vi "Main Flir-Ax8.vi"() -> ()   [LabVIEW 2016]
uses:
  X-Control/Run.xctl
  <vilib>/vision/Image Controls.llb/IMAQ Image.ctl
  Global Flir-Ax8.vi
  <vilib>/httpClient/LabVIEWHTTPClient.lvlib
panel:
  out "live temperature":dbl format="%#_3g"
  out "Active":bool
  in  "Tab Control":enum32{"initialize", "Thermal", "Data"}(tab)
  in  "Password :":string="admin"
  in  "User Name :":string="admin"
  in  "IP Address :":string="169.254.60.23"
  in  "File name & format :":string="Thermal.csv"
  in  "Image Folder :":path=path "C:/Users/Matanel/Desktop/Final Project/project versions/Flir-Ax8"
  in  "Run":dbl(xcontrol)
  out "Image":T1(plugin-control)
  in  "Stop":bool
  out "High Temperature":bool
  out "Temperature In Range":bool
  in  "Take image":bool
  out "Temperature":cluster{dbl, dbl, dbl, dbl, dbl}(slide)={0.0, 12.0, 13.0, 0.0, 0.0} scale=0.0..60.0 scale format="%#_3g"
  in  "Temperature Limit":dbl=60.0
  in  "Min Temperature":dbl=15.0
  in  "Max Temperature":dbl=60.0
  out "Communication":bool
  in  "Reset":bool
  in  "Table":string[][](table)
  # "Flir-Ax8 Thermal Image"
  # "11"
  # "8"
  # "1"
  # "1"
  # "3"
  # "4"
  # "3"
  # "6"
  # "1"
  # "2"
  # "1"
  # "4"
  # "Login"
  # "Initialize Data"
  # "9"
  # "10"
  # "5"
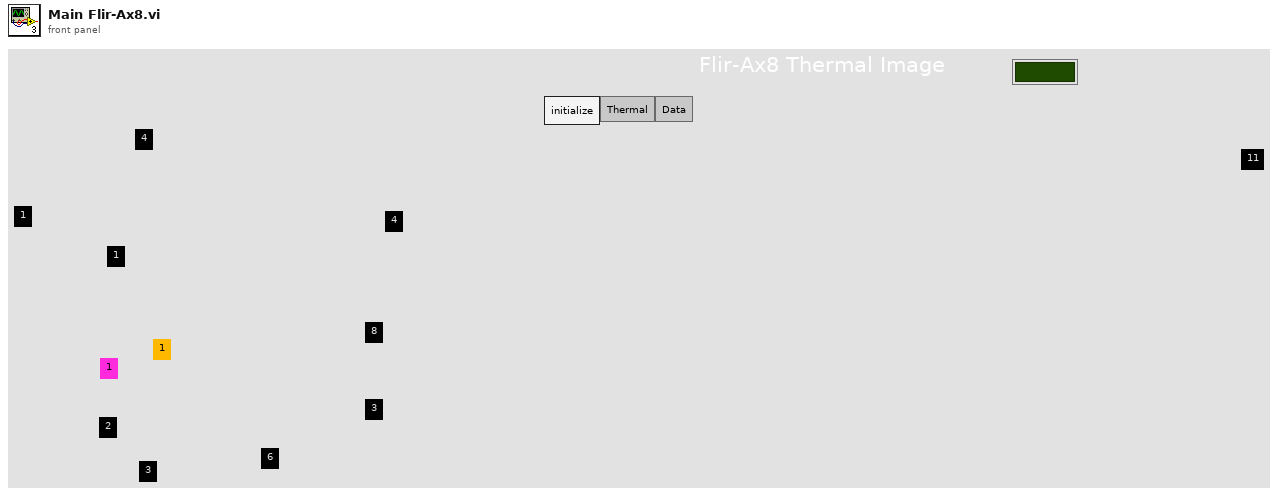
[diagram p1: front panel]
types:
  T1 = typedef "IMAQ Image.ctl" = refnum<image>
  T2 = enum8{"Enabled", "Disabled", "Disabled and Grayed Out"}
  T3 = typedef "imagedata.ctl" = cluster{"image type":i32, "image depth":i32, "image":u8[], "mask":u8[], "colors":u32[], "Rectangle":cluster{"left":i16, "top":i16, "right":i16, "bottom":i16}}
  T4 = typedef "Image Type" = u32
  T5 = typedef "LabVIEWHTTPClient.lvlib/ClientHandle.ctl" = refnum<k1>
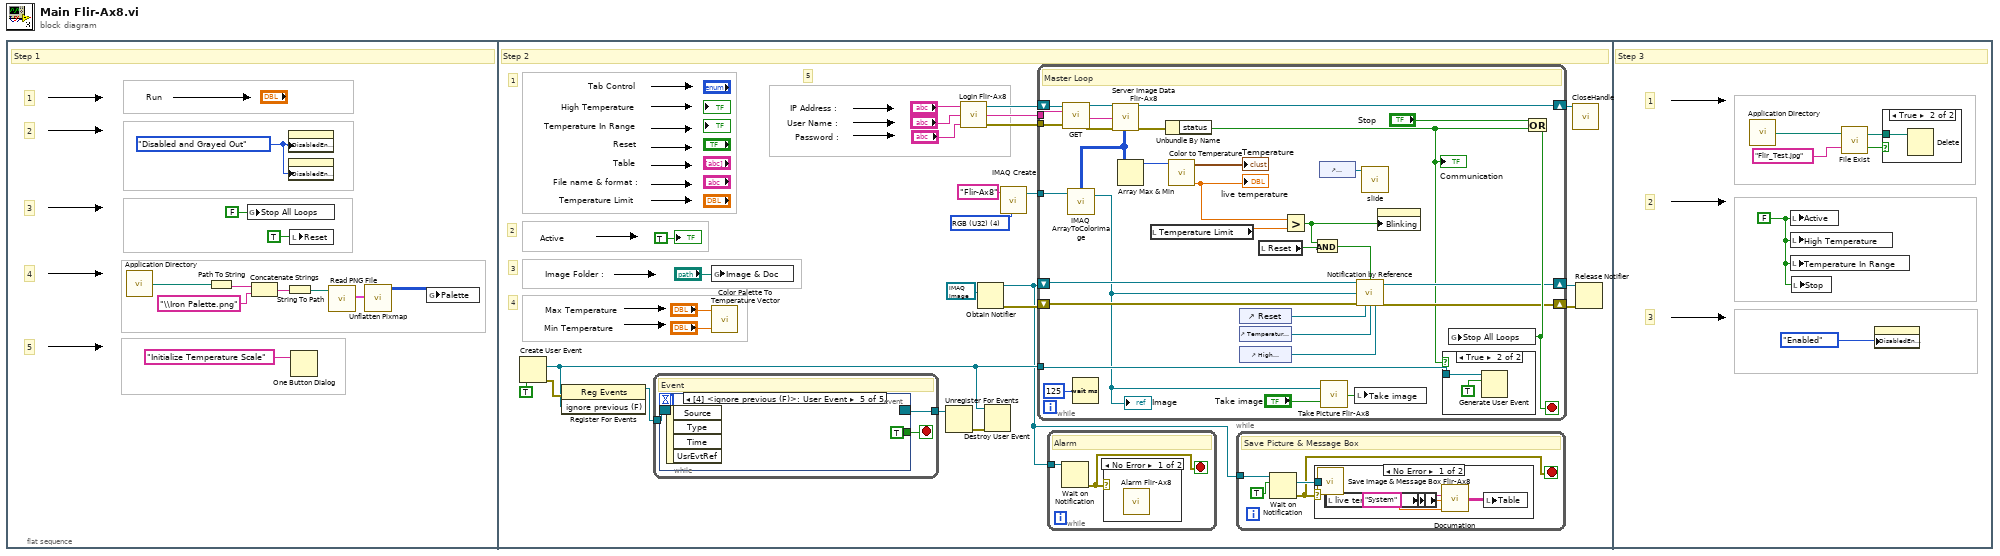
[diagram p0: block diagram]
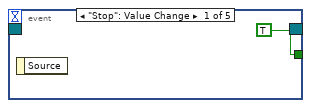
[diagram p2: hidden frame]
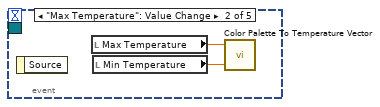
[diagram p3: hidden frame]
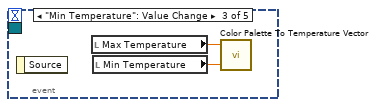
[diagram p4: hidden frame]
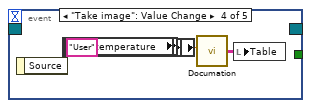
[diagram p5: hidden frame]
diagram:
  n1 = flat-sequence {
    frame #0 {
      w1 = T2."Disabled and Grayed Out" ("Disabled")
      # "5"
      # "4"
      # "3"
      # "2"
      # "1"
      # "Step 1"
      n2 = call <vilib>:"Application Directory.vi"() -> ("Application Directory"=w2:path)
      n3 = Path To String(path=w2) -> (string=w6:string)
      n4 = global write "Global Flir-Ax8.vi" "Stop All Loops"(FALSE ("Stop All Loops")) -> ()
      n5 = Concatenate Strings ("add")(w6, "\\Iron Palette.png" ("string")) -> (w5:string)
      n6 = String To Path(string=w5) -> (path=w4:path)
      n7 = property on="Run" class="Run (strict)"("DisabledEnum"=w1) -> ()  [unwired: 2 in, 2 out]
      n8 = property on="Reset" class="Bool (strict)"("DisabledEnum"=w1) -> ()  [unwired: 2 in, 2 out]
      n9 = local write "Reset"(TRUE ("Reset")) -> ()
      n10 = One Button Dialog(message="Initialize Temperature Scale") -> ()  [unwired: 1 in, 1 out]
      n11 = call <vilib>:"Read PNG File.vi"("path to PNG file"=w4) -> ("image data"=w10:T3)  [unwired: 8 in, 2 out]
      n12 = call <vilib>:"Unflatten Pixmap.vi"("image data"=w10) -> ("24-bit pixmap"=w11:u32[][])  [unwired: 4 in, 6 out]
      n13 = global write "Global Flir-Ax8.vi" "Palette"(w11) -> ()
    }
    frame #1 {
      w35 = T4 4 items=["Grayscale (U8)", "Grayscale (I16)", "Grayscale (SGL)", "Complex (CSG)", "RGB (U32)", "HSL (U32)", "RGB (U64)", "Grayscale (U16)"] ("Image Type")
      # "5"
      # "4"
      # "3"
      # "2"
      # "1"
      # "Step 2"
      n14 = Create User Event(user event datatype=TRUE ("ignore previous (F)")) -> (user event=w13:refnum<user-event>, error out=w23:errorcluster)  [unwired: 1 in]
      n15 = register-events(error in=w23, w13) -> (reference out=w21:refnum<event-registration>)  [unwired: 1 in, 1 out]
      n16 = while {
        tunnel: w21 -> [w39]
        tunnel: [w38] -> w20
        stop <- w37 stop-if-true
        # "Event"
        n17 = event shown="[4] <ignore previous (F)>: User Event" {
          selector: w39 -> [_ _ _ _ _]
          dyn-events: [_ _ _ _ _] -> w38
          timeout: _ -> [_ _ _ _ _]
          tunnel: [TRUE ("Active") _ _ _ TRUE ("Active")] -> w37
          event "Stop": Value Change {
            n18 = event-data() -> ()  [unwired: 1 in, 1 out]
          }
          event "Max Temperature": Value Change {
            n19 = event-data() -> ()  [unwired: 1 in, 1 out]
            n20 = local read "Max Temperature"() -> (w42:dbl)
            n21 = local read "Min Temperature"() -> (w41:dbl)
            n22 = call "Color Palette To Temperature Vector.vi"("Min Temperature"=w41, "Max Temperature"=w42) -> ()  [unwired: 3 in]
          }
          event "Min Temperature": Value Change {
            n23 = event-data() -> ()  [unwired: 1 in, 1 out]
            n24 = local read "Max Temperature"() -> (w44:dbl)
            n25 = local read "Min Temperature"() -> (w43:dbl)
            n26 = call "Color Palette To Temperature Vector.vi"("Min Temperature"=w43, "Max Temperature"=w44) -> ()  [unwired: 3 in]
          }
          event "Take image": Value Change {
            n27 = event-data() -> ()  [unwired: 1 in, 1 out]
            n28 = local read "Min Temperature"() -> (w49:dbl)
            n29 = local read "File name & format :"() -> (w46:string)
            n30 = local read "live temperature"() -> (w47:dbl)
            n31 = local read "Max Temperature"() -> (w50:dbl)
            n32 = call "Documation.vi"("Max Scale"=w50, "File Nm and format"=w46, "User/System"="User" ("File Nm and format"), "Temp"=w47, "Min Scale"=w49) -> ("Table"=w45:string[][])
            n33 = local write "Table"(w45) -> ()
          }
          event User Event {
            n34 = event-data() -> ()  [unwired: 1 in, 4 out]
          }
        }
      }
      n35 = global write "Global Flir-Ax8.vi" "Image & Doc"("Image Folder :") -> ()
      n36 = call "Color Palette To Temperature Vector.vi"("Min Temperature"="Min Temperature", "Max Temperature"="Max Temperature") -> ()  [unwired: 3 in]
      n37 = Unregister For Events(event registration refnum=w20) -> (error out=w19:errorcluster)  [unwired: 1 in]
      n38 = call "Login Flir-Ax8.vi"("Password"="Password :", "User Name"="User Name :", "IP"="IP Address :") -> ("Error"=w24:errorcluster, "Image Request"=w31:string, "Client Handle"=w32:T5)
      n39 = Obtain Notifier(notification data type=T1 refnum ("Image Out")) -> (notifier out=w12:refnum<notifier>, error out=w18:errorcluster)  [unwired: 2 in, 2 out]
      n40 = Destroy User Event(user event=w13, error in=w19) -> ()  [unwired: 1 out]
      n41 = call "IMAQ Create"("Image Name"="Flir-Ax8", "Image Type"=w35) -> ("New Image"=w33:T1)  [unwired: 3 in, 1 out]
      n42 = while {
        shift-right: [w81] -> w26
        shift-left: w18 -> [w79]
        shift-right: [w82] -> w27
        shift-left: w12 -> [w80]
        shift-right: [w94] -> w25
        shift-left: w32 -> [w95]
        tunnel: w33 -> [w93]
        tunnel: w31 -> [w92]
        tunnel: w24 -> [w88]
        tunnel: w13 -> [w68]
        stop <- w83 stop-if-true
        # "Master Loop"
        n43 = call <vilib>:"GET.vi"("client handle"=w95, "url"=w92, "error in (no error)"=w88) -> ("client handle out"=w94:T5, "body"=w73:string, "error out"=w72:errorcluster)  [unwired: 9 in, 1 out]
        n44 = Wait (ms)(milliseconds to wait=u32 125) -> ()  [unwired: 1 out]
        n45 = call "Server Image Data Flir-Ax8.vi"("Server Data"=w73, "Error In"=w72) -> ("Image matrix out"=w86:u32[][], "Error Out"=w87:errorcluster)  [unwired: 12 in]
        n46 = call "IMAQ ArrayToColorImage"("Image Pixels (U32)"=w86, "Image"=w93) -> ("Image Out"=w67:T1)  [unwired: 3 in, 1 out]
        "Image" <- w67
        n47 = Array Max & Min(array=w86) -> (max value=w74:u32)  [unwired: 3 out]
        n48 = local read "Temperature Limit"() -> (w85:dbl)
        n49 = Unbundle By Name(w87) -> ("status"=w65:bool)
        "Communication" <- w65
        n50 = call "Color to Temperature.vi"("Color"=w74) -> ("Temperature"=w70:dbl, "Slide"=→"Temperature":cluster{dbl, dbl, dbl, dbl, dbl})  [unwired: 7 in]
        "live temperature" <- w70
        n51 = control-ref of="Reset"() -> (w77:refnum<vi>)
        n52 = control-ref of="Temperature In Range"() -> (w76:refnum<vi>)
        n53 = control-ref of="High Temperature"() -> (w75:refnum<vi>)
        n54 = local read "Reset"() -> (w84:bool)
        n55 = Greater?(x=w70, y=w85) -> (0:w69:bool)
        n56 = And(x=w69, y=w84) -> (x .and. y?=w78:bool)
        n57 = control-ref of="Temperature"() -> (w90:refnum<vi>)
        n58 = call "Take Picture Flir-Ax8.vi"("Take Picture"="Take image", "Image"=w67) -> ("Reset Button"=w89:bool)
        n59 = local write "Take image"(w89) -> ()
        n60 = call "Notification by Reference.vi"("Notifier In"=w80, "Temperature & Reset"=w78, "Image In"=w67, "Error In"=w79, "Reset"=w77, "Temperature In Range"=w76, "High Temperature"=w75) -> ("Notifier out"=w82:refnum<notifier>, "Error out"=w81:errorcluster)  [unwired: 7 in]
        n61 = call "slide.vi"("Slide in"=w90) -> ()  [unwired: 11 in]
        n62 = property on="Temperature" class="Slide (strict)"("Blinking"=w69) -> ()  [unwired: 2 in, 2 out]
        n63 = case shown="True" w65 {
          tunnel: w68 -> [_ w97]
          frame False {
          }
          frame True {
            n64 = Generate User Event(user event=w97, event data cluster=TRUE ("ignore previous (F)")) -> ()  [unwired: 2 in, 2 out]
          }
        }
        n65 = Or(x="Stop", y=w65) -> (x .or. y?=w83:bool)
        n66 = global write "Global Flir-Ax8.vi" "Stop All Loops"(w83) -> ()
      }
      n67 = while {
        tunnel: w12 -> [w63]
        stop <- w64 stop-if-true
        # "Alarm"
        n68 = Wait on Notification(notifier=w63) -> (error out=w64:errorcluster)  [unwired: 1 in, 5 out]
        n69 = case shown="No Error" w64 {
          frame No Error {
            n70 = call "Alarm Flir-Ax8.vi"() -> ()  [unwired: 2 in]
          }
          frame Error {
          }
        }
      }
      n71 = while {
        tunnel: w12 -> [w52]
        stop <- w53 stop-if-true
        # "Save Picture & Message Box"
        n72 = Wait on Notification(notifier=w52, ignore previous (F)=TRUE) -> (notification=w55:T1, error out=w53:errorcluster)  [unwired: 1 in, 3 out]
        n73 = case shown="No Error" w53 {
          tunnel: w55 -> [w62 _]
          frame No Error {
            n74 = call "Save Image & Message Box Flir-Ax8.vi"("Image"=w62) -> ()  [unwired: 1 in]
            n75 = local read "File name & format :"() -> (w57:string)
            n76 = local read "Max Temperature"() -> (w60:dbl)
            n77 = local read "live temperature"() -> (w61:dbl)
            n78 = local read "Min Temperature"() -> (w59:dbl)
            n79 = call "Documation.vi"("Max Scale"=w60, "File Nm and format"=w57, "User/System"="System" ("File Nm and format"), "Temp"=w61, "Min Scale"=w59) -> ("Table"=w56:string[][])
            n80 = local write "Table"(w56) -> ()
          }
          frame Error {
          }
        }
      }
      n81 = call <vilib>:"CloseHandle.vi"("client handle"=w25) -> ()  [unwired: 14 in, 1 out]
      n82 = Release Notifier(notifier=w27, error in (no error)=w26) -> ()  [unwired: 4 out]
      "Active" <- TRUE ("Boolean")
    }
    frame #2 {
      w99 = FALSE ("Active")
      # "3"
      # "2"
      # "1"
      # "Step 3"
      n83 = call <vilib>:"Application Directory.vi"() -> ("Application Directory"=w102:path)
      n84 = local write "Active"(w99) -> ()
      n85 = local write "High Temperature"(w99) -> ()
      n86 = local write "Temperature In Range"(w99) -> ()
      n87 = local write "Stop"(w99) -> ()
      n88 = call "File Exist.vi"("File Nm"="Flir_Test.jpg", "File path"=w102) -> ("File Exists"=w104:bool, "Appended path"=w103:path)
      n89 = property on="Run" class="Run (strict)"("DisabledEnum"=T2."Enabled" ("Disabled")) -> ()  [unwired: 2 in, 2 out]
      n90 = case shown="True" w104 {
        tunnel: w103 -> [_ w105]
        frame False {
        }
        frame True {
          n91 = Delete(path (use dialog)=w105) -> ()  [unwired: 4 in, 3 out]
        }
      }
    }
  }
